vi "Modbus_writing.vi"() -> ()   [LabVIEW 2019]
uses:
  <vilib>/NI/Modbus Library/API/Wrapper/Create Serial Master.vi
  <vilib>/NI/Modbus Library/API/Master/Modbus Master.lvclass
  <vilib>/NI/Modbus Library/API/Wrapper/API Main.lvlib
panel:
  out "Voltaje VFD":dbl
  out "Corriente VFD":dbl
  out "Corriente VFD":dbl(knob) scale=0.0..2.0
  out "Voltaje VFD":dbl(knob) scale=0.0..220.0
  in  "VFD":bool
  in  "Baud rate":u32=9600
  in  "Puerto":refnum<visa-resource-name>
  in  "stop":bool
  in  "Frequency":dbl(knob) step=1.0 scale=0.0..75.0
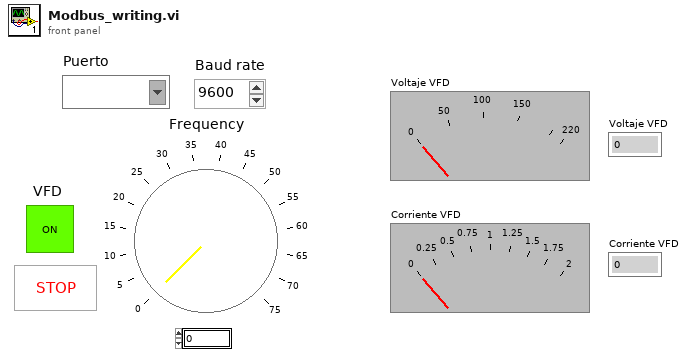
[diagram p1: front panel]
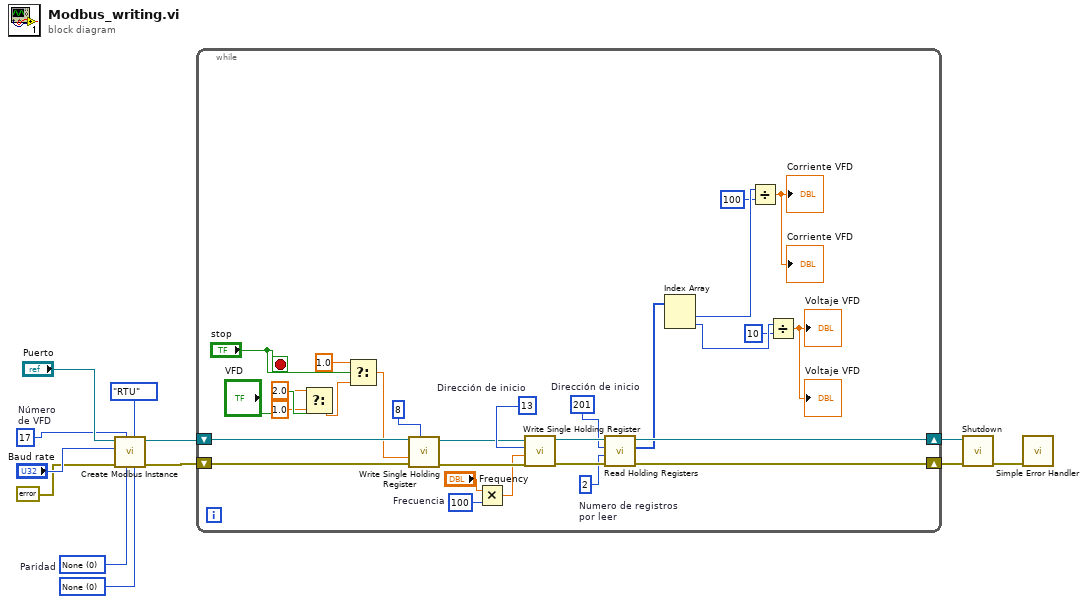
[diagram p0: block diagram]
diagram:
  w2 = u16 0 items=["None", "Odd", "Even", "Mark", "Space"]  # Paridad
  w3 = u16 0 items=["None", "XON/XOFF", "RTS/CTS", "XON/XOFF & RTS/CTS", "DTR/DSR", "XON/XOFF & DTR/DSR"] ("flow control (none)")
  w1 = u8 17  # Número de VFD
  n1 = call-poly <vilib>:"Create Modbus Instance.vi"("flow control (none)"=w3, "serial type"=enum16{"RTU", "ASCII"}."RTU", "parity (even)"=w2, "unit ID"=w1, "error in"=errorcluster {"status"=FALSE, "code"=0, "source"=""}, "baud rate"="Baud rate", "VISA resource name"="Puerto") -> ("error out"=w10:errorcluster, "serial master instance"=w12:refnum<class "Modbus Master.lvclass">)  [unwired: 3 in]
  n2 = while {
    shift-right: [w21] -> w11
    shift-left: w12 -> [w40]
    shift-right: [w20] -> w9
    shift-left: w10 -> [w41]
    stop <- "stop" stop-if-true
    w22 = u16 2  # Numero de registros  por leer
    w23 = u16 201  # Dirección de inicio
    w31 = u16 100  # Frecuencia
    w38 = u16 13  # Dirección de inicio
    n3 = Select(t=2.0, s="VFD", f=1.0) -> (s? t:f=w27:dbl)
    n4 = Select(t=1.0, s="stop", f=w27) -> (s? t:f=w28:dbl)
    n5 = call-dynamic "Write Single Holding Register.vi"("error in"=w41, "register to write"=w28, "address"=u16 8 ("Start"), "Modbus master in"=w40) -> ("error out"=w36:errorcluster, "Modbus master out"=w37:refnum<class "Modbus Master.lvclass">)  [unwired: 6 in]
    n6 = Multiply(x="Frequency", y=w31) -> (x*y=w30:dbl)
    n7 = call-dynamic "Write Single Holding Register.vi"("error in"=w36, "register to write"=w30, "address"=w38, "Modbus master in"=w37) -> ("error out"=w24:errorcluster, "Modbus master out"=w25:refnum<class "Modbus Master.lvclass">)  [unwired: 6 in]
    n8 = call-dynamic "Read Holding Registers.vi"("error in"=w24, "number of inputs"=w22, "starting address"=w23, "Modbus master in"=w25) -> ("error out"=w20:errorcluster, "register values"=w19:u16[], "Modbus master out"=w21:refnum<class "Modbus Master.lvclass">)  [unwired: 5 in]
    n9 = Index Array(array=w19) -> (element #1=w15:u16, element #2=w18:u16)  [unwired: 2 in]
    n10 = Divide(x=w15, y=u16 100) -> (x/y=→"Corriente VFD" →"Corriente VFD":dbl)
    n11 = Divide(x=w18, y=u16 10) -> (x/y=→"Voltaje VFD" →"Voltaje VFD":dbl)
  }
  n12 = call-dynamic "Shutdown.vi"("error in"=w9, "Modbus master in"=w11) -> ("error out"=w4:errorcluster)  [unwired: 9 in]
  n13 = call <vilib>:"Simple Error Handler.vi"("error in (no error)"=w4) -> ()  [unwired: 4 in, 5 out]
